vi "SetTxPower.vi"(6 "Legacy (f)?":bool, 8 "error in (no error)":errorcluster, 10 "TxPower":dbl[](array[numeric]) format="%.2f") -> (0 "error out":errorcluster)   [LabVIEW 2011]
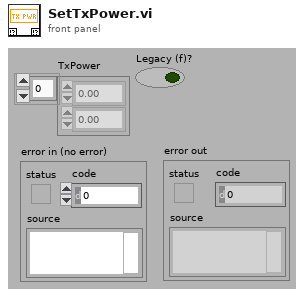
[diagram p1: front panel]
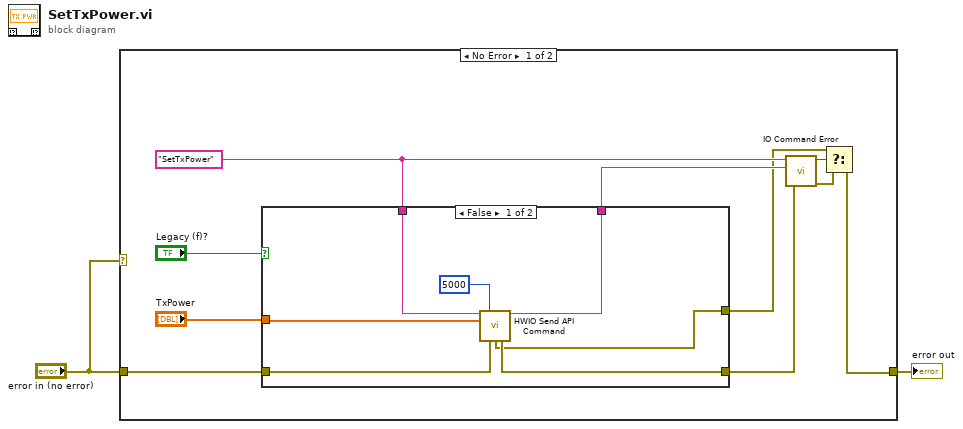
[diagram p0: block diagram]
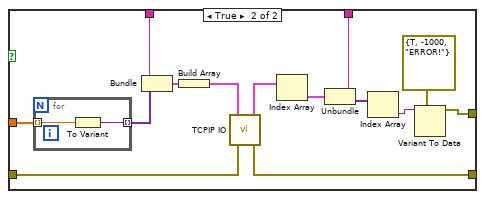
[diagram p2: hidden frame]
diagram:
  n1 = case shown="No Error" "error in (no error)" {
    tunnel: "error in (no error)" -> [w11 w36]
    tunnel: [w5 w36] -> w2
    frame No Error {
      w9 = "SetTxPower"
      n2 = case shown="False" "Legacy (f)?" {
        tunnel: "TxPower" -> [w15 w33]
        tunnel: w11 -> [w19 w31]
        tunnel: [w18 w29] -> w10
        tunnel: w9 -> [w16 w28]
        tunnel: [w17 w25] -> w8
        tunnel: [w14 w20] -> w4
        frame False {
          n3 = call "HWIO Send API Command.vi"("Action"=w16, "Timeout ms (5000)"=5000 ("PerCommand Timeout (ms)"), "Double"=w15, "error in (no error)"=w19) -> ("Action out"=w17:string, "HWError"=w14:errorcluster, "error out"=w18:errorcluster)  [unwired: 4 in, 5 out]
        }
        frame True {
          n4 = for {
            tunnel: w33 -> [w35] mode=indexing
            tunnel: [w34] -> w32 mode=indexing
            n5 = To Variant(anything=w35) -> (Variant=w34:variant)
          }
          n6 = Bundle(w28, w32) -> (w30:cluster{string, variant[]})  [unwired: 1 out]
          n7 = Build Array(w30) -> (w24:cluster{string, variant[]}[])
          n8 = call "TCPIP IO.vi"("error in (no error)"=w31, "Commands"=w24) -> ("error out"=w29:errorcluster, "Responses"=w26:cluster{string, variant[]}[])  [unwired: 1 in, 3 out]
          n9 = Index Array(array=w26) -> (element=w27:cluster{string, variant[]})  [unwired: 1 in]
          n10 = Unbundle(w27) -> (w25:string, w21:variant[])
          n11 = Index Array(array=w21) -> (element=w23:variant)  [unwired: 1 in]
          n12 = Variant To Data(type=errorcluster {"status"=TRUE, "code"=-1000, "source"="ERROR!"} ("error out"), Variant=w23) -> (data=w20:errorcluster)  [unwired: 1 in, 1 out]
        }
      }
      n13 = call "IO Command Error.vi"("error in (no error)"=w10, "Command Returned (\"\")"=w8, "Command Sent (\"\")"=w9) -> ("error out"=w6:errorcluster, "HW ERR?"=w7:bool)  [unwired: 3 out]
      n14 = Select(t=w4, s=w7, f=w6) -> (s? t:f=w5:errorcluster)
    }
    frame Error {
    }
  }
  "error out" <- w2
